vi "Dequeue Message.vi"(7 "timeout in ms (-1)":i32=-1, 11 "channel":T1) -> (1 "message data":variant, 2 "message":string, 3 "timed out?":bool)   [LabVIEW 2023, in "Message Queue.lvlib"]
doc: "This VI takes messages out of the messenger channel."
uses:
  Message Queue.lvlib
  <extravilib>/ChannelInstances/Messenger-t'Message Queue.lvlib-Message Cluster.ctl'/))Channel.ctl
  Message Cluster.ctl
  <extravilib>/ChannelInstances/Messenger-t'Message Queue.lvlib-Message Cluster.ctl'/Read With Abort.vi
  <extravilib>/ChannelInstances/Messenger-t'Message Queue.lvlib-Message Cluster.ctl'/Endpoint.vi
  <extravilib>/ChannelInstances/Messenger-t'Message Queue.lvlib-Message Cluster.ctl'.lvlib
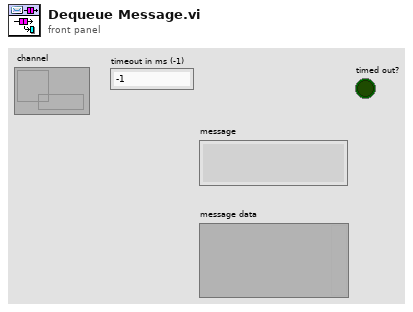
[diagram p1: front panel]
types:
  T1 = typedef "Messenger-t'Message Queue.lvlib-Message Cluster.ctl'.lvlib/))Channel.ctl" = refnum<queue>
  T2 = typedef "Message Queue.lvlib/Message Cluster.ctl" = cluster{"Message":string, "Message Data":variant}
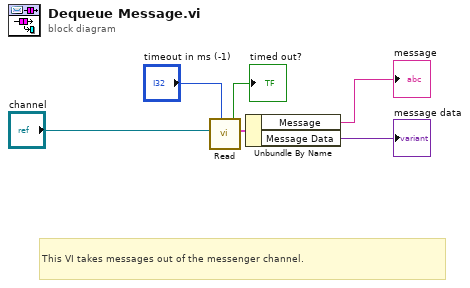
[diagram p0: block diagram]
diagram:
  # "This VI takes messages out of the messenger channel."
  n1 = call <extravilib>:"Read.vi"("timeout in ms (-1)"="timeout in ms (-1)", "channel"="channel") -> ("element"=w6:T2, "timed out?"=→"timed out?":bool)  [unwired: 7 in, 1 out]
  n2 = Unbundle By Name(w6) -> ("Message"=→"message":string, "Message Data"=→"message data":variant)
